vi "find_index.vi"(8 "error in (no error)":errorcluster, 10 "ID":dbl, 11 "PointCollection in":refnum<class "PointCollection.lvclass">) -> (0 "error out":errorcluster, 1 "found?":bool, 2 "index":i32, 3 "PointCollection out":refnum<class "PointCollection.lvclass">)   [LabVIEW 2010, in "PointCollection.lvclass"]
uses:
  PointCollection.lvclass
  mode_enum.ctl
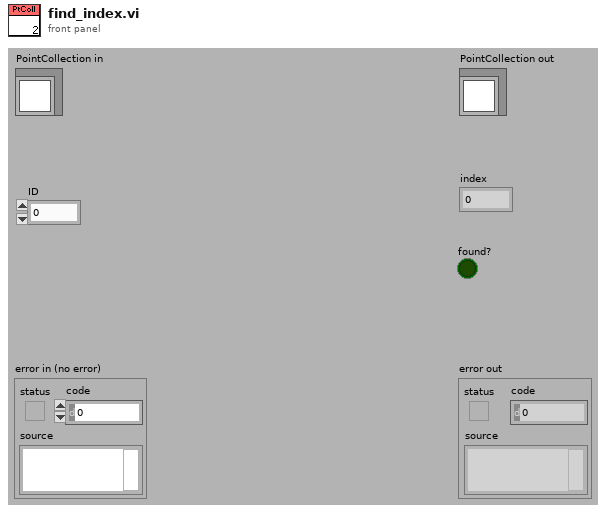
[diagram p1: front panel]
types:
  T1 = typedef "PointCollection.lvclass/mode_enum.ctl" = enum16{"points first", "dimensions first"}
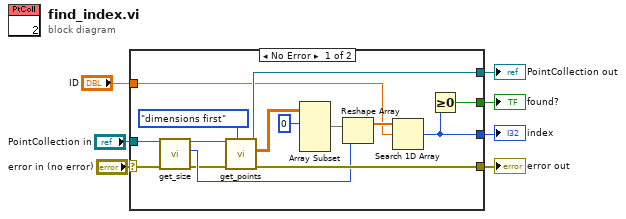
[diagram p0: block diagram]
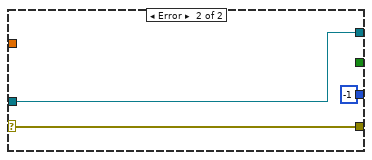
[diagram p2: hidden frame]
diagram:
  n1 = case shown="No Error" "error in (no error)" {
    selector: "error in (no error)" -> [w8 w25]
    tunnel: [w22 w25] -> w6
    tunnel: [w20 w24] -> w4
    tunnel: "PointCollection in" -> [w12 w24]
    tunnel: "ID" -> [w15 _]
    tunnel: [w14 -1 ("index of element")] -> w2
    tunnel: [w13 _] -> w1
    frame No Error {
      n2 = call "get_size.vi"("error in (no error)"=w8, "PointCollection in"=w12) -> ("error out"=w9:errorcluster, "number of points"=w11:i32, "PointCollection out"=w10:refnum<class "PointCollection.lvclass">)  [unwired: 7 in]
      n3 = call-dynamic "get_points.vi"("retrieval mode"=mode_enum."dimensions first", "error in (no error)"=w9, "PointCollection in"=w10) -> ("error out"=w22:errorcluster, "points"=w19:dbl[][], "PointCollection out"=w20:refnum<class "PointCollection.lvclass">)  [unwired: 6 in]
      n4 = Array Subset(array=w19, index (row)=0 ("index")) -> (w17:dbl[][])  [unwired: 3 in]
      n5 = Reshape Array(w17, w11) -> (w16:dbl[])
      n6 = Search 1D Array(1D array=w16, element=w15) -> (index of element=w14:i32)  [unwired: 1 in]
      n7 = Greater Or Equal To 0?(x=w14) -> (x >= 0?=w13:bool)
    }
    frame Error {
    }
  }
  "error out" <- w6
  "PointCollection out" <- w4
  "index" <- w2
  "found?" <- w1
